vi "M Solar cells.vi"(11 "EV3 in":T1) -> (3 "EV3 out":T1)   [LabVIEW 2016]
uses:
  <vilib>/NXT/Subs/LVHSConnector.ctl
  <vilib>/NXT/LegoClasses/BrickReference/BrickReference.lvclass
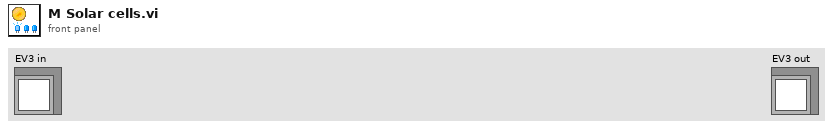
[diagram p1: front panel]
types:
  T1 = typedef "LVHSConnector.ctl" = refnum<class "BrickReference.lvclass">
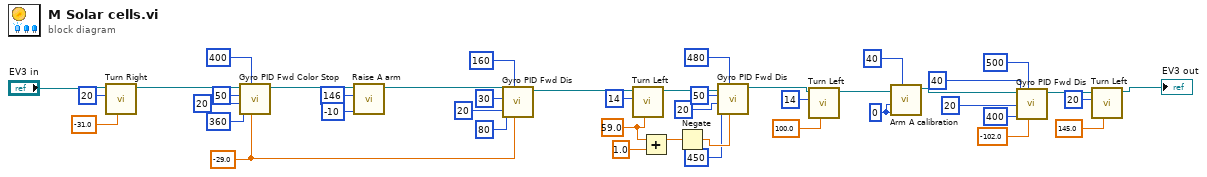
[diagram p0: block diagram]
diagram:
  w12 = i8 0 ("Down Power")
  w23 = sgl 59.0 ("Turning angle")
  w29 = sgl -29.0 ("Target angle")
  n1 = call "Turn Right.vi"("Turning angle"=sgl -31.0, "Motor B (right)"=i8 20, "EV3 in"="EV3 in") -> ("EV3 out"=w43:T1)  [unwired: 8 in]
  n2 = call "Gyro PID Fwd Color Stop.vi"("Target angle"=w29, "Threshold to Color"=400 ("Threshold to stop"), "Threshold to slow"=360, "Min. speed"=20, "Max. speed"=50, "EV3 in"=w43) -> ("EV3 out"=w36:T1)  [unwired: 5 in]
  n3 = call "Raise A arm.vi"("Power"=i8 -10, "Rotation"=146, "EV3 in"=w36) -> ("EV3 out"=w30:T1)  [unwired: 8 in]
  n4 = call "Gyro PID Fwd Dis.vi"("Target angle"=w29, "Threshold to stop"=160, "Threshold to slow"=80, "Min. speed"=20, "Max. speed"=30, "EV3 in"=w30) -> ("EV3 out"=w28:T1)  [unwired: 5 in]
  n5 = call "Turn Left.vi"("Turning angle"=w23, "Motor B (right)"=i8 14, "EV3 in"=w28) -> ("EV3 out"=w26:T1)  [unwired: 8 in]
  n6 = Add(x=w23, y=sgl 1.0) -> (x+y=w22:sgl)
  n7 = Negate(x=w22) -> (-x=w20:sgl)
  n8 = call "Gyro PID Fwd Dis.vi"("Target angle"=w20, "Threshold to stop"=480, "Threshold to slow"=450, "Min. speed"=20, "Max. speed"=50, "EV3 in"=w26) -> ("EV3 out"=w16:T1)  [unwired: 5 in]
  n9 = call "Turn Left.vi"("Turning angle"=sgl 100.0, "Motor B (right)"=i8 14, "EV3 in"=w16) -> ("EV3 out"=w13:T1)  [unwired: 8 in]
  n10 = call "Arm A calibration.vi"("Cali. Power"=i8 40, "Down Power"=w12, "Rotation"=w12, "NXT/EV3"=w13) -> ("NXT/EV3"=w10:T1)  [unwired: 7 in]
  n11 = call "Gyro PID Fwd Dis.vi"("Target angle"=sgl -102.0, "Threshold to stop"=500, "Threshold to slow"=400, "Min. speed"=20, "Max. speed"=40, "EV3 in"=w10) -> ("EV3 out"=w4:T1)  [unwired: 5 in]
  n12 = call "Turn Left.vi"("Turning angle"=sgl 145.0, "Motor B (right)"=i8 20, "EV3 in"=w4) -> ("EV3 out"=→"EV3 out":T1)  [unwired: 8 in]
